vi "Stop Data Stream.vi"(8 "error in (no error)":errorcluster, 11 "Statnett C37.118 DLL in":refnum<class "Statnett C37.118 DLL.lvclass">) -> (0 "error out":errorcluster, 3 "Statnett C37.118 DLL out":refnum<class "Statnett C37.118 DLL.lvclass">)   [LabVIEW 2013, in "PMU Recorder Light.lvlib" / "Statnett C37.118 DLL.lvclass"]
uses:
  Statnett C37.118 DLL.lvclass
  Statnett C37.118 DLL.lvclass/Statnett C37.118 DLL.ctl
  c37118-dll/labview/C37118-DLL.lvlib
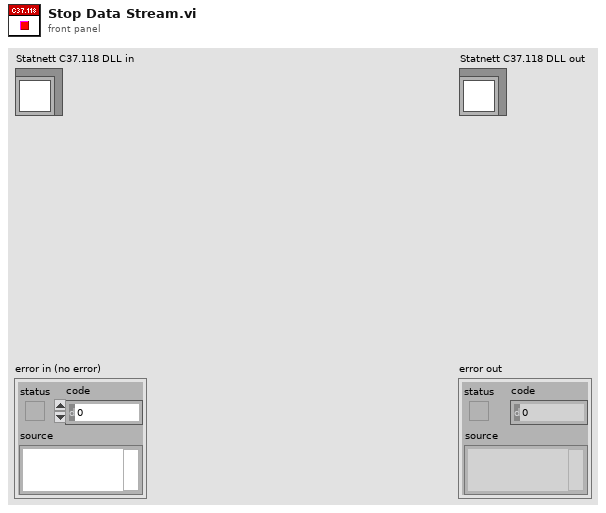
[diagram p1: front panel]
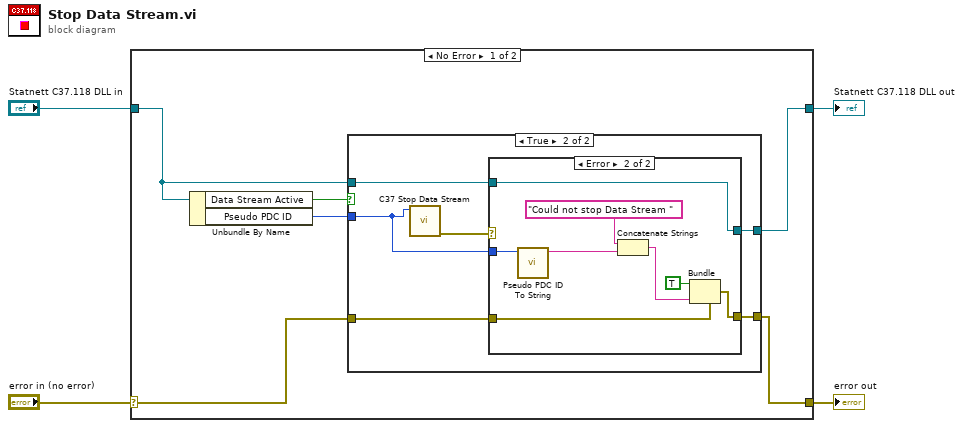
[diagram p0: block diagram]
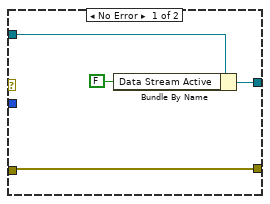
[diagram p3: hidden frame]
diagram:
  n1 = case shown="No Error" "error in (no error)" {
    selector: "error in (no error)" -> [w6 w32]
    tunnel: [w5 w32] -> w3
    tunnel: [w7 w31] -> w1
    tunnel: "Statnett C37.118 DLL in" -> [w8 w31]
    frame No Error {
      n2 = Unbundle By Name(w8) -> ("Data Stream Active"=w9:bool, "Pseudo PDC ID"=w10:i32)
      n3 = case shown="True" w9 {
        tunnel: w10 -> [_ w14]
        tunnel: w8 -> [w12 w18]
        tunnel: [w12 w17] -> w7
        tunnel: w6 -> [w11 w16]
        tunnel: [w11 w15] -> w5
        frame False {
        }
        frame True {
          n4 = call "C37 Stop Data Stream.vi"("Pseudo PDC ID"=w14) -> ("error out"=w13:errorcluster)  [unwired: 10 in]
          n5 = case shown="Error" w13 {
            tunnel: w18 -> [w22 w26]
            tunnel: [w20 w26] -> w17
            tunnel: w14 -> [_ w25]
            tunnel: w16 -> [w19 w24]
            tunnel: [w19 w23] -> w15
            frame No Error {
              n6 = Bundle By Name(cluster=w22, "Data Stream Active"=FALSE) -> (w20:refnum<class "Statnett C37.118 DLL.lvclass">)
            }
            frame Error {
              n7 = call "Pseudo PDC ID To String.vi"("Pseudo PDC ID"=w25) -> ("String"=w27:string)  [unwired: 10 in]
              n8 = Concatenate Strings("Could not stop Data Stream " ("source"), w27) -> (w30:string)
              n9 = Bundle(cluster=w24, "status"=TRUE, "source"=w30) -> (w23:errorcluster)  [unwired: 1 in]
            }
          }
        }
      }
    }
    frame Error {
    }
  }
  "error out" <- w3
  "Statnett C37.118 DLL out" <- w1
